vi "3654Turbo.vi"(10 "ButtonPressed?":bool, 11 "Input":dbl) -> (3 "Output":dbl)   [LabVIEW 2017]
uses:
  Robot Global Data.vi
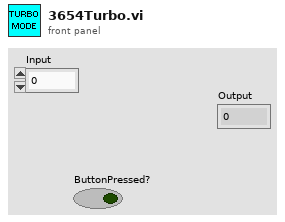
[diagram p1: front panel]
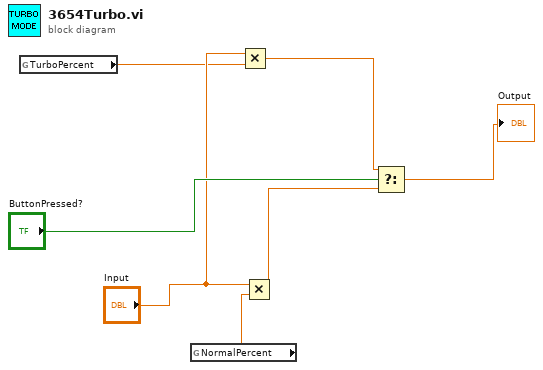
[diagram p0: block diagram]
diagram:
  n1 = global read "Robot Global Data.vi" "TurboPercent"() -> (w2:dbl)
  n2 = global read "Robot Global Data.vi" "NormalPercent"() -> (w1:dbl)
  n3 = Multiply(x="Input", y=w2) -> (x*y=w4:dbl)
  n4 = Multiply(x="Input", y=w1) -> (x*y=w6:dbl)
  n5 = Select(t=w4, s="ButtonPressed?", f=w6) -> (s? t:f=→"Output":dbl)
